vi "ServiceClient.vi"(0 "Msg in":string, 2 "Topic":string="/junk", 3 "node":string) -> (4 "Reply":string)   [LabVIEW 2012]
doc: "Starts a service client on the RIO"
uses:
  <userlib>/ROSforLV/ROS/Code/Console/Servers/ServerSubs/TopicDef.ctl
  <userlib>/ROSforLV/ROS/Code/SubVIs/_ROSDirection.ctl
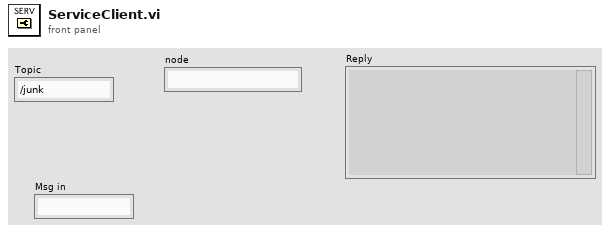
[diagram p1: front panel]
types:
  T1 = typedef "TopicDef.ctl" = cluster{"Topic":string, "Type":string, "Action":T2, "Update (ms)":u16, "queue size":u16}
  T2 = typedef "_ROSDirection.ctl" = enum16{"Node", "Publisher", "Subscriber", "Service Client"}
  T3 = typedef "_ROSControl.ctl" = cluster{"topic port":u16, "Node":string, "topic":string, "type":string, "node port":u16, "error ":errorcluster, "Direction":T2, "Update (ms)":u16, "queue size":u16}
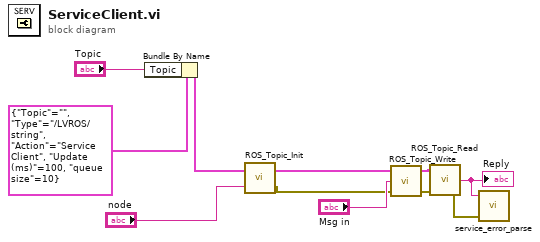
[diagram p0: block diagram]
diagram:
  n1 = Bundle By Name(cluster=T1 {"Topic"="", "Type"="/LVROS/string", "Action"=enum."Service Client", "Update (ms)"=100, "queue size"=10} ("Definitions"), "Topic"="Topic") -> (w5:T1)
  n2 = call <userlib>:"ROS_Topic_Init.vi"("node"="node", "Definitions"=w5) -> ("error out"=w3:errorcluster, "ROS out"=w9:T3)
  n3 = call <userlib>:"ROS_Topic_Write.vi"("error in (no error)"=w3, "Msg in"="Msg in", "ROS in"=w9) -> ("error out"=w2:errorcluster, "ROS out"=w10:T3)  [unwired: 1 in]
  n4 = call <userlib>:"ROS_Topic_Read.vi"("error in (no error)"=w2, "ROS in"=w10) -> ("error out"=w1:errorcluster, "Reply"=w11:string)  [unwired: 1 in, 1 out]
  "Reply" <- w11
  n5 = call <userlib>:"service_error_parse.vi"("error in (no error)"=w1, "Reply"=w11) -> ()  [unwired: 1 in, 3 out]
